vi "Get Object by Class name.vi"(8 "error in (no error)":errorcluster, 10 "Class name":string, 11 "Cache Manager DVR in":refnum<class "Cache Manager.lvclass">) -> (0 "error out":errorcluster, 2 "Serialize out":refnum<class "Serializable Msg.lvclass">, 3 "Cache Manager DVR out":refnum<class "Cache Manager.lvclass">)   [LabVIEW 2020, in "Cache Manager.lvclass"]
uses:
  Cache Manager.lvclass
  Serializer/Serializable Message/Serializable Msg.lvclass
  Cache Manager.lvclass/Cache Manager.ctl
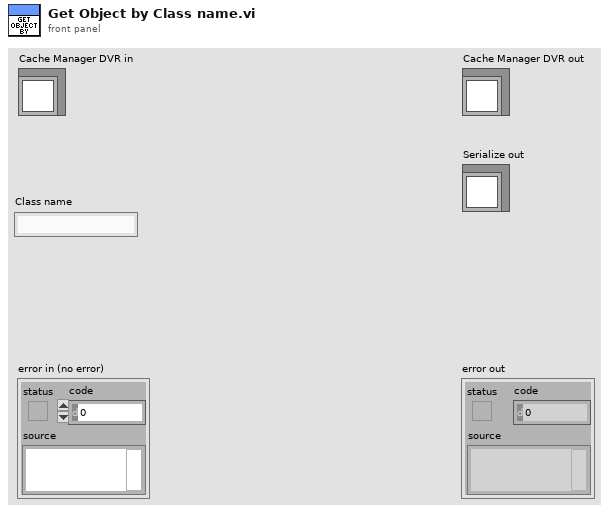
[diagram p1: front panel]
types:
  T1 = map{string, refnum<class "Serializable Msg.lvclass">}
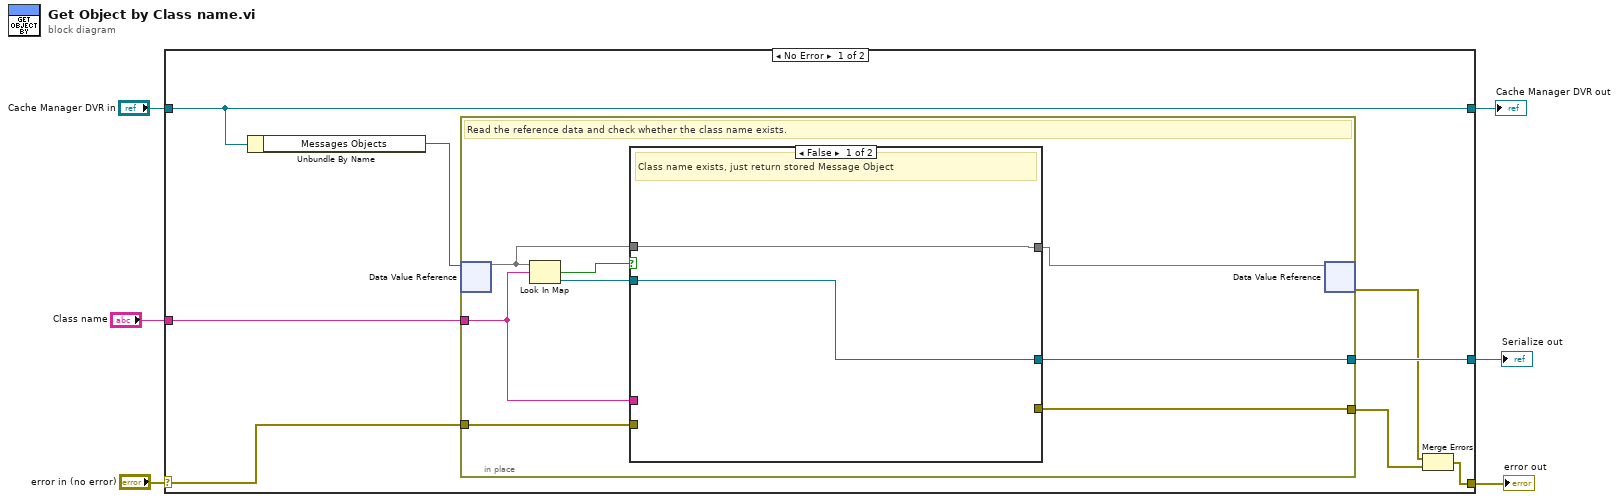
[diagram p0: block diagram]
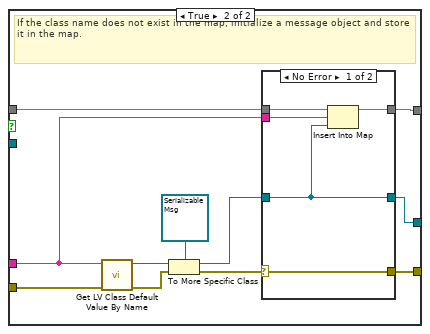
[diagram p2: hidden frame]
diagram:
  n1 = case shown="No Error" "error in (no error)" {
    selector: "error in (no error)" -> [w7 w43]
    tunnel: [w10 w43] -> w5
    tunnel: [w14 w42] -> w3
    tunnel: "Cache Manager DVR in" -> [w14 w42]
    tunnel: "Class name" -> [w12 _]
    tunnel: [w11 _] -> w1
    frame No Error {
      n2 = Unbundle By Name(w14) -> ("Messages Objects"=w13:refnum<data-value>)
      n3 = in-place {
        in-place-border: w12 -> [w21]
        in-place-border: [w18] -> w11
        in-place-border: [w16] -> w8
        in-place-border: w7 -> [w15]
        # "Read the reference data and check whether the class name exists."
        n4 = in-place-dvr #1(w13) -> (w20:T1)  [unwired: 1 out]
        n5 = Look In Map(map=w20, key=w21) -> (key not found?=w22:bool, value=w19:refnum<class "Serializable Msg.lvclass">)  [unwired: 1 in]
        n6 = case shown="False" w22 {
          tunnel: [w23 w32] -> w17
          tunnel: w21 -> [_ w30]
          tunnel: w20 -> [w23 w31]
          tunnel: w19 -> [w24 _]
          tunnel: [w24 w27] -> w18
          tunnel: [_ w26] -> w16
          tunnel: w15 -> [_ w25]
          frame False {
            # "Class name exists, just return stored Message Object"
          }
          frame True {
            # "If the class name does not exist in the map, initialize a message object and store it in the map."
            n7 = call <vilib>:"Get LV Class Default Value By Name.vi"("error in (no error)"=w25, "class name"=w30) -> ("error out"=w35:errorcluster, "object"=w33:refnum<class>)  [unwired: 8 in]
            n8 = To More Specific Class(target class=refnum<class "Serializable Msg.lvclass"> refnum ("Serializable Message.lvclass"), reference=w33, error in=w35) -> (specific class reference=w29:refnum<class "Serializable Msg.lvclass">, error out=w28:errorcluster)
            n9 = case shown="No Error" w28 {
              selector: w28 -> [w36 w41]
              tunnel: [w40 _] -> w32
              tunnel: w31 -> [w39 _]
              tunnel: w30 -> [w38 _]
              tunnel: w29 -> [w37 _]
              tunnel: [w37 _] -> w27
              tunnel: [w36 w41] -> w26
              frame No Error {
                n10 = Insert Into Map(map in=w39, key=w38, value=w37) -> (map out=w40:T1)  [unwired: 2 out]
              }
              frame Error {
                # "If it is not possible to instantiate the object for any reason, do not store an empty object."
              }
            }
          }
        }
        n11 = in-place-dvr #1(w17) -> (w9:errorcluster)  [unwired: 1 out]
      }
      n12 = Merge Errors(w9, w8) -> (w10:errorcluster)
    }
    frame Error {
    }
  }
  "error out" <- w5
  "Cache Manager DVR out" <- w3
  "Serialize out" <- w1
